vi "Action Update Ramp Rate.vi"(8 "error in (no error)":errorcluster, 11 "Temperature Ramp Rate":dbl) -> (0 "error out":errorcluster)   [LabVIEW 2015, in "Thermal Chamber Controller_DQMH.lvlib"]
uses:
  Thermal Chamber Controller_DQMH.lvlib
  Thermal Chamber Response Simulator/Thermal Chamber Response Simulator.lvlib
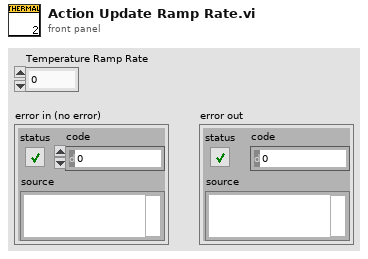
[diagram p1: front panel]
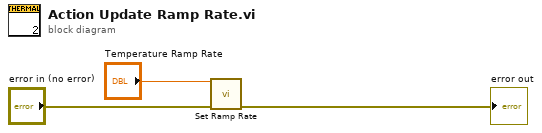
[diagram p0: block diagram]
diagram:
  n1 = call "Set Ramp Rate.vi"("error in (no error)"="error in (no error)", "Ramp Rate (deg C / second)"="Temperature Ramp Rate") -> ("error out"=→"error out":errorcluster)  [unwired: 9 in]
